vi "FTW-Ether-NewLoggerConnection.vi"(5 "Logger Address":string, 11 "error in":errorcluster) -> (4 "Event Logger Connection":refnum<class "FTW-Logger.lvclass">, 15 "error out":errorcluster)   [LabVIEW 2013, in "FTW-Ether.lvclass"]
uses:
  FTW-Ether.lvclass
  EventLogger/FTW-Logger.lvclass
  FTW-Ether-Instance.vi
panel:
  # "Inputs"
  # "Outputs"
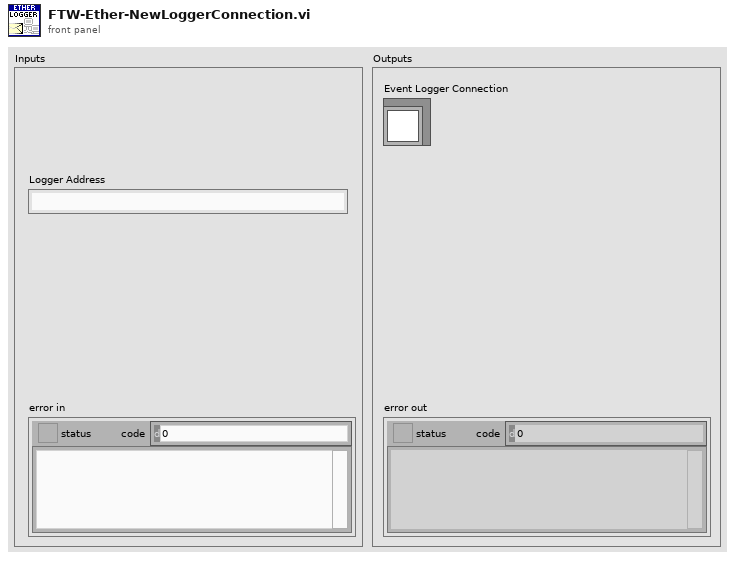
[diagram p1: front panel]
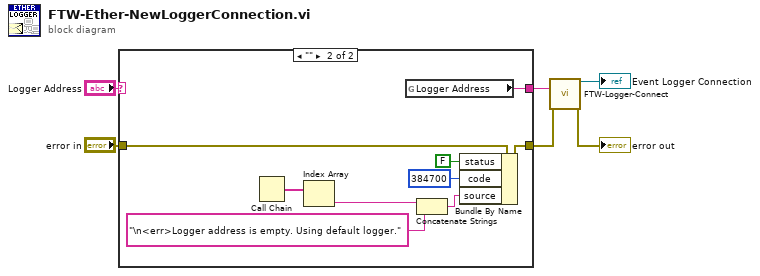
[diagram p0: block diagram]
diagram:
  n1 = case shown="\"\"" "Logger Address" {
    selector: "Logger Address" -> [w8 _]
    tunnel: [w8 w17] -> w4
    tunnel: "error in" -> [w7 w16]
    tunnel: [w7 w15] -> w1
    frame Default {
    }
    frame "" {
      n2 = Call Chain() -> (call chain=w10:string[])
      n3 = Index Array(array=w10) -> (element=w9:string)  [unwired: 1 in]
      n4 = global read "FTW-Ether-Instance.vi" "Logger Address"() -> (w17:string)
      n5 = Concatenate Strings(w9, "\n<err>Logger address is empty. Using default logger." ("Warning Message")) -> (w11:string)
      n6 = Bundle By Name(cluster=w16, "status"=FALSE, "code"=384700 ("Error Code"), "source"=w11) -> (w15:errorcluster)
    }
  }
  n7 = call "FTW-Logger-Connect.vi"("Logger Address"=w4, "error in"=w1) -> ("FTW Logger Connector"=→"Event Logger Connection":refnum<class "FTW-Logger.lvclass">, "error out"=→"error out":errorcluster)  [unwired: 12 in]
